vi "Translate Wheel.vi"(8 "error in (no error)":errorcluster, 9 "new position":cluster{"x":dbl, "y":dbl}, 10 "wheel index":i32, 11 "steering frame ref in":refnum<data-value>) -> (0 "error out":errorcluster, 3 "steering frame ref out":refnum<data-value>)   [LabVIEW 2017, in "NI_Robotics_Configure Steering Frame.lvlib"]
uses:
  <vilib>/robotics/Dialog/Configure Steering Frame/NI_Robotics_Configure Steering Frame.lvlib
  <vilib>/robotics/Steering/Steering Frame/NI_Robotics_Steering Frame.lvclass
  <vilib>/robotics/Steering/Differential Steering Frame/NI_Robotics_Differential Steering Frame.lvclass
  c:/Program Files (x86)/National Instruments/LabVIEW 2017/vi.lib/robotics/Steering/Steering Frame/NI_Robotics_Steering Frame.lvclass
  <vilib>/robotics/Steering/Steering Frame/NI_Robotics_Steering Frame.lvclass/NI_Robotics_Steering Frame.ctl
  <vilib>/robotics/Steering/Wheel/NI_Robotics_Wheel.lvclass/NI_Robotics_Wheel.ctl
  <vilib>/robotics/Steering/Differential Steering Frame/NI_Robotics_Differential Steering Frame.lvclass/NI_Robotics_Differential Steering Frame.ctl
  <vilib>/robotics/Steering/Ackermann Steering Frame/NI_Robotics_Ackermann Steering Frame.lvclass
  <vilib>/robotics/Steering/Ackermann Steering Frame/NI_Robotics_Ackermann Steering Frame.lvclass/NI_Robotics_Ackermann Steering Frame.ctl
  <vilib>/robotics/Steering/Mecanum Steering Frame/NI_Robotics_Mecanum Steering Frame.lvclass
  <vilib>/robotics/Steering/Mecanum Steering Frame/NI_Robotics_Mecanum Steering Frame.lvclass/NI_Robotics_Mecanum Steering Frame.ctl
  <vilib>/robotics/Steering/Differential Steering Frame/Set Wheel Separation.vi
  <vilib>/robotics/Steering/Ackermann Steering Frame/Get Wheel Separations.vi
  <vilib>/robotics/Steering/Ackermann Steering Frame/Set Wheel Separations.vi
  <vilib>/robotics/Steering/Mecanum Steering Frame/Set Wheel Separations.vi
  <vilib>/robotics/Steering/Differential Steering Frame/Wheel Separation to Frame Positions.vi
  <vilib>/robotics/Steering/Steering Frame/Reposition Wheels.vi
  <vilib>/robotics/Steering/Ackermann Steering Frame/Wheel Separation to Frame Positions.vi
  <vilib>/robotics/Steering/Mecanum Steering Frame/Wheel Separation to Frame Positions.vi
  <vilib>/robotics/Steering/Wheel/Update Steering to Wheel Frame Transform.vi
  <vilib>/Analysis/coordinate.llb/Wrap Angle.vi
  <vilib>/Analysis/coordinate.llb/Wrap Angle (scalar).vi
  <vilib>/robotics/Steering/Steering Frame/Reposition Single Wheel on Steering Frame.vi
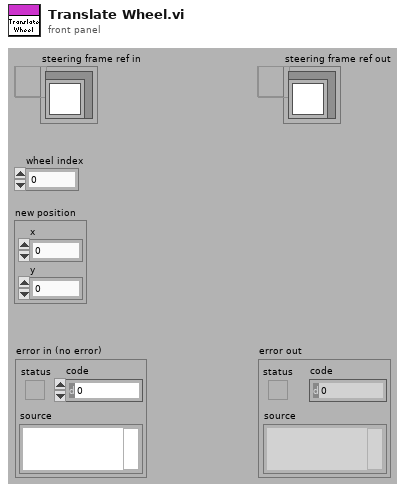
[diagram p1: front panel]
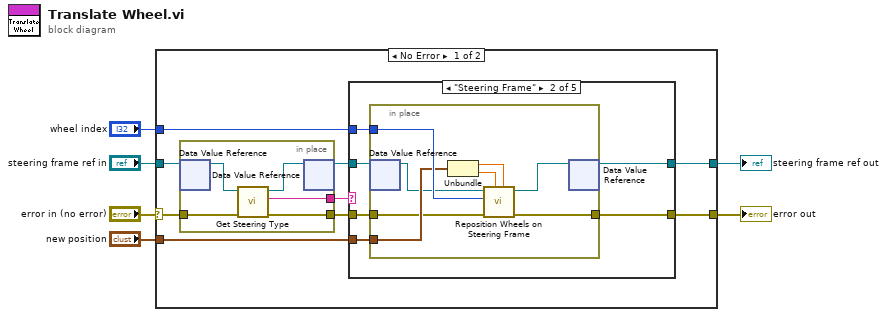
[diagram p0: block diagram]
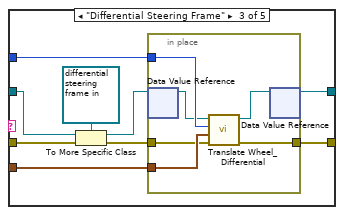
[diagram p3: hidden frame]
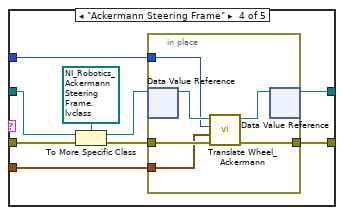
[diagram p4: hidden frame]
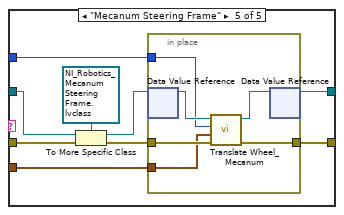
[diagram p5: hidden frame]
diagram:
  n1 = case shown="No Error" "error in (no error)" {
    selector: "error in (no error)" -> [w15 w83]
    tunnel: [w12 w83] -> w5
    tunnel: "wheel index" -> [w11 _]
    tunnel: "new position" -> [w10 _]
    tunnel: "steering frame ref in" -> [w9 w82]
    tunnel: [w7 w82] -> w1
    frame No Error {
      n2 = in-place {
        in-place-border: w15 -> [w20]
        in-place-border: [w19] -> w14
        in-place-border: [w18] -> w13
        n3 = in-place-dvr #1(w9) -> (w17:refnum<class "NI_Robotics_Steering Frame.lvclass">)  [unwired: 1 out]
        n4 = call-dynamic "Get Steering Type.vi"("error in (no error)"=w20, "steering frame in"=w17) -> ("error out"=w18:errorcluster, "steering type"=w19:string, "steering frame out"=w16:refnum<class "NI_Robotics_Steering Frame.lvclass">)  [unwired: 7 in]
        n5 = in-place-dvr #1(w16) -> (w8:refnum<data-value>)  [unwired: 1 out]
      }
      n6 = case shown="\"Steering Frame\"" w14 {
        tunnel: w13 -> [w22 w26 w45 w60 w75]
        tunnel: [w22 w25 w44 w59 w74] -> w12
        tunnel: w11 -> [_ w28 w42 w57 w72]
        tunnel: w10 -> [_ w27 w43 w58 w73]
        tunnel: w8 -> [w21 w24 w40 w55 w70]
        tunnel: [w21 w23 w37 w52 w67] -> w7
        frame Default {
        }
        frame "Steering Frame" {
          n7 = in-place {
            in-place-border: w28 -> [w34]
            in-place-border: w27 -> [w33]
            in-place-border: w26 -> [w32]
            in-place-border: [w31] -> w25
            n8 = in-place-dvr #2(w24) -> (w30:refnum<class "NI_Robotics_Steering Frame.lvclass">)  [unwired: 1 out]
            n9 = Unbundle(w33) -> ("x"=w36:dbl, "y"=w35:dbl)
            n10 = call-poly <vilib>:"Reposition Wheels on Steering Frame.vi"("x position"=w36, "y position"=w35, "error in (no error)"=w32, "wheel index"=w34, "steering frame in"=w30) -> ("error out"=w31:errorcluster, "steering frame out"=w29:refnum<class "NI_Robotics_Steering Frame.lvclass">)  [unwired: 4 in, 1 out]
            n11 = in-place-dvr #2(w29) -> (w23:refnum<data-value>)  [unwired: 1 out]
          }
        }
        frame "Differential Steering Frame" {
          n12 = To More Specific Class(target class=refnum<data-value> refnum ("steering frame ref in"), reference=w40, error in=w45) -> (specific class reference=w38:refnum<data-value>, error out=w41:errorcluster)
          n13 = in-place {
            in-place-border: [w51] -> w44
            in-place-border: w43 -> [w50]
            in-place-border: w42 -> [w49]
            in-place-border: w41 -> [w48]
            n14 = in-place-dvr #3(w38) -> (w47:refnum<class "NI_Robotics_Differential Steering Frame.lvclass">)  [unwired: 1 out]
            n15 = call <vilib>:"Translate Wheel_Differential.vi"("error in (no error)"=w48, "new position"=w50, "wheel index"=w49, "differential steering frame in"=w47) -> ("error out"=w51:errorcluster, "differantial steering frame out"=w46:refnum<class "NI_Robotics_Differential Steering Frame.lvclass">)  [unwired: 6 in]
            n16 = in-place-dvr #3(w46) -> (w37:refnum<data-value>)  [unwired: 1 out]
          }
        }
        frame "Ackermann Steering Frame" {
          n17 = To More Specific Class(target class=refnum<data-value> refnum ("steering frame ref in"), reference=w55, error in=w60) -> (specific class reference=w53:refnum<data-value>, error out=w56:errorcluster)
          n18 = in-place {
            in-place-border: [w63] -> w59
            in-place-border: w58 -> [w61]
            in-place-border: w57 -> [w62]
            in-place-border: w56 -> [w64]
            n19 = in-place-dvr #4(w53) -> (w66:refnum<class "NI_Robotics_Ackermann Steering Frame.lvclass">)  [unwired: 1 out]
            n20 = call <vilib>:"Translate Wheel_Ackermann.vi"("error in (no error)"=w64, "new position"=w61, "wheel index"=w62, "ackermann steering frame in"=w66) -> ("error out"=w63:errorcluster, "ackermann steering frame out"=w65:refnum<class "NI_Robotics_Ackermann Steering Frame.lvclass">)  [unwired: 6 in]
            n21 = in-place-dvr #4(w65) -> (w52:refnum<data-value>)  [unwired: 1 out]
          }
        }
        frame "Mecanum Steering Frame" {
          n22 = To More Specific Class(target class=refnum<data-value> refnum ("steering frame ref in"), reference=w70, error in=w75) -> (specific class reference=w68:refnum<data-value>, error out=w71:errorcluster)
          n23 = in-place {
            in-place-border: [w78] -> w74
            in-place-border: w73 -> [w76]
            in-place-border: w72 -> [w77]
            in-place-border: w71 -> [w79]
            n24 = in-place-dvr #5(w68) -> (w81:refnum<class "NI_Robotics_Mecanum Steering Frame.lvclass">)  [unwired: 1 out]
            n25 = call <vilib>:"Translate Wheel_Mecanum.vi"("error in (no error)"=w79, "new position"=w76, "wheel index"=w77, "mecanum steering frame in"=w81) -> ("error out"=w78:errorcluster, "mecanum steering frame out"=w80:refnum<class "NI_Robotics_Mecanum Steering Frame.lvclass">)  [unwired: 6 in]
            n26 = in-place-dvr #5(w80) -> (w67:refnum<data-value>)  [unwired: 1 out]
          }
        }
      }
    }
    frame Error {
    }
  }
  "error out" <- w5
  "steering frame ref out" <- w1
